vi "Loop Calculation Function.vi"(3 "Number of Steps":string="0") -> (0 "No. of Scan Points":i32, 1 "Remainder":string)   [LabVIEW 2020]
doc: "Calculates the number of scanning points along 1 axis for the raster scan. Each scan point is 1mm (5000 steps) away from each other which is why the total number of steps is divided by 5000 to give the number of scan points. \n\nArgs:\n\nNumber of Steps: Input as a a string as the output to 'Distance To Steps.vi' is a string\n\nReturns:\n\nNo. of Scan Points: The total number of scans that need to occur along 1 axis\nRemainder: The remaining steps from the calculation which the machine still needs to perform to ensure it has covered the entire distance of the scanning tank."
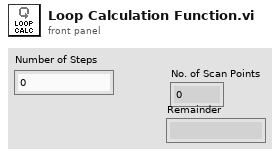
[diagram p1: front panel]
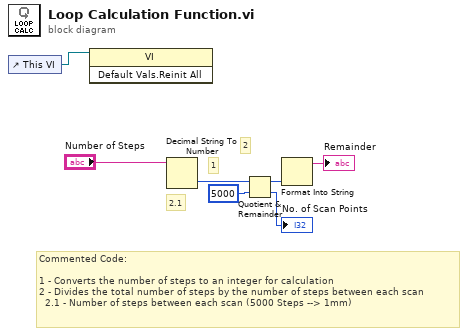
[diagram p0: block diagram]
diagram:
  # "2.1"
  # "2"
  # "1"
  # "Commented Code:\n\n1 - Converts the number of steps to an integer for calculation\n2 - Divides the total number of steps by the number of steps between each scan\n  2.1 - Number of steps between each scan (5000 Steps --> 1mm)"
  n1 = control-ref of="This VI"() -> (w1:refnum<vi>)
  n2 = invoke class="VI" method="Default Vals.Reinit All"(reference=w1) -> ()  [unwired: 2 in, 3 out]
  n3 = Decimal String To Number(string="Number of Steps") -> (number=w6:i32)  [unwired: 2 in, 1 out]
  n4 = Quotient & Remainder(x=w6, y=5000) -> (x-y*floor(x/y)=w3:i32, floor(x/y)=→"No. of Scan Points":i32)
  n5 = Format Into String(w3) -> (resulting string=→"Remainder":string)  [unwired: 3 in, 1 out]
